vi "Convert PID Parameters.vi"(4 "Derivative Unit":enum16{"min", "s"}(ring), 5 "Proportional Unit":enum16{"Gain (Kc)", "Band (PB)"}(ring)=enum."Band (PB)", 6 "Integral Unit":enum16{"min", "s"}(ring), 7 "PID Structure":T2(ring), 9 "Derivative":dbl, 10 "Integral":dbl, 11 "Proportional":dbl) -> (3 "PID gains":T1)   [LabVIEW 2023]
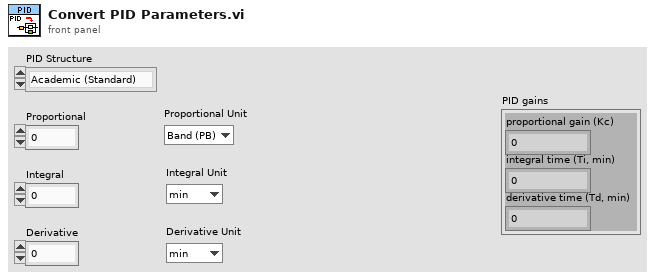
[diagram p1: front panel]
types:
  T1 = cluster{"proportional gain (Kc)":dbl, "integral time (Ti, min)":dbl, "derivative time (Td, min)":dbl}
  T2 = enum16{"Academic (Standard)", "Parallel", "Series"}
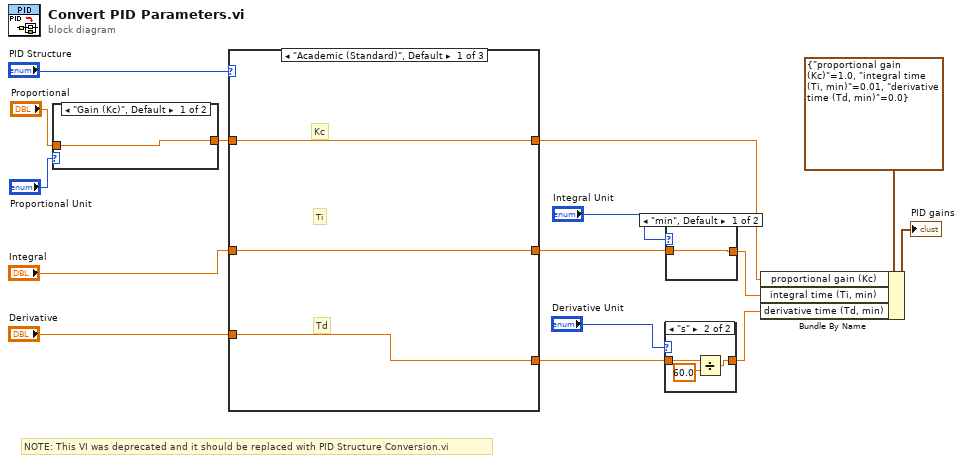
[diagram p0: block diagram]
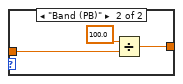
[diagram p2: hidden frame]
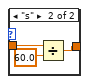
[diagram p4: hidden frame]
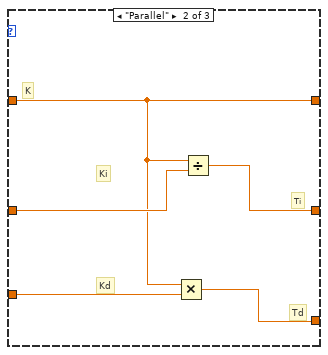
[diagram p5: hidden frame]
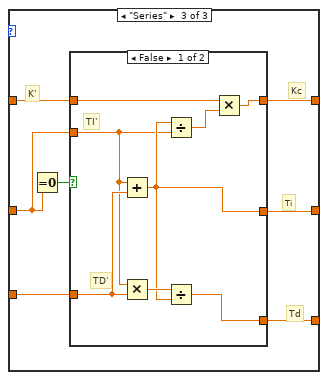
[diagram p6: hidden frame]
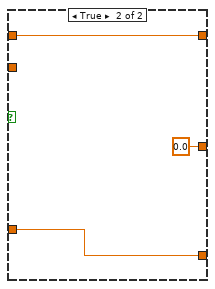
[diagram p7: hidden frame]
diagram:
  # "NOTE: This VI was deprecated and it should be replaced with PID Structure Conversion.vi"
  n1 = case shown="\"Gain (Kc)\", Default" "Proportional Unit" {
    tunnel: "Proportional" -> [w16 w17]
    tunnel: [w16 w19] -> w2
    frame "Gain (Kc)", Default {
    }
    frame "Band (PB)" {
      n2 = Divide(x=100.0, y=w17) -> (x/y=w19:dbl)
    }
  }
  n3 = case shown="\"Academic (Standard)\", Default" "PID Structure" {
    tunnel: "Derivative" -> [w22 w25 w32]
    tunnel: "Integral" -> [w21 w27 w28]
    tunnel: [w22 w23 w30] -> w6
    tunnel: [w21 w26 w31] -> w5
    tunnel: [w20 w24 w33] -> w1
    tunnel: w2 -> [w20 w24 w34]
    frame "Academic (Standard)", Default {
      # "Td"
      # "Ti"
      # "Kc"
    }
    frame "Parallel" {
      # "Td"
      # "Ti"
      # "Kd"
      # "Ki"
      # "K"
      n4 = Multiply(x=w24, y=w25) -> (x*y=w23:dbl)
      n5 = Divide(x=w24, y=w27) -> (x/y=w26:dbl)
    }
    frame "Series" {
      # "K'"
      # "Td"
      # "Kc"
      # "Ti"
      n6 = Equal To 0?(x=w28) -> (x = 0?=w29:bool)
      n7 = case shown="False" w29 {
        tunnel: w34 -> [w42 w45]
        tunnel: [w40 w45] -> w33
        tunnel: w32 -> [w39 w43]
        tunnel: [w37 0.0] -> w31
        tunnel: [w36 w43] -> w30
        tunnel: w28 -> [w35 _]
        frame False {
          # "TD'"
          # "TI'"
          n8 = Add(x=w35, y=w39) -> (x+y=w37:dbl)
          n9 = Multiply(x=w35, y=w39) -> (x*y=w38:dbl)
          n10 = Divide(x=w37, y=w35) -> (x/y=w41:dbl)
          n11 = Divide(x=w38, y=w37) -> (x/y=w36:dbl)
          n12 = Multiply(x=w42, y=w41) -> (x*y=w40:dbl)
        }
        frame True {
        }
      }
    }
  }
  n13 = case shown="\"s\"" "Derivative Unit" {
    tunnel: w6 -> [w46 w49]
    tunnel: [w46 w47] -> w7
    frame "min", Default {
    }
    frame "s" {
      n14 = Divide(x=w49, y=60.0) -> (x/y=w47:dbl)
    }
  }
  n15 = case shown="\"min\", Default" "Integral Unit" {
    tunnel: w5 -> [w50 w53]
    tunnel: [w50 w51] -> w8
    frame "min", Default {
    }
    frame "s" {
      n16 = Divide(x=w53, y=60.0) -> (x/y=w51:dbl)
    }
  }
  n17 = Bundle By Name(cluster=T1 {"proportional gain (Kc)"=1.0, "integral time (Ti, min)"=0.01, "derivative time (Td, min)"=0.0} ("PID gains"), "proportional gain (Kc)"=w1, "integral time (Ti, min)"=w8, "derivative time (Td, min)"=w7) -> (→"PID gains":T1)
